vi "Reboot Target.vi"(8 "Error In":errorcluster, 11 "Install LV Data":T1={"SSH Session"=refnum, "Status Log"="", "Detailed Log"="", "Credentials"={"Hostname or IP"="192.168.7.2", "Username"="root", "Password"=""}, "Target Info"={"OS Version"="", "CPU"="", "Systemd Version"="", "Internet Access"=FALSE, "Device Type"="", "LV Installed Ver"="", "LV Available Ver"="", "LV Upgrade Available"=FALSE, "Hostname"="", "NIC Info"=[]}, "Reboot Required?"=FALSE}) -> (0 "Error Out":errorcluster, 1 "Connected?":bool, 3 "Install LV Data":T1={"SSH Session"=refnum, "Status Log"="", "Detailed Log"="", "Credentials"={"Hostname or IP"="192.168.7.2", "Username"="root", "Password"=""}, "Target Info"={"OS Version"="", "CPU"="", "Systemd Version"="", "Internet Access"=FALSE, "Device Type"="", "LV Installed Ver"="", "LV Available Ver"="", "LV Upgrade Available"=FALSE, "Hostname"="", "NIC Info"=[]}, "Reboot Required?"=FALSE})   [LabVIEW 2020, in "LMH-LINX.lvlib"]
uses:
  LMH-LINX.lvlib
  Target Management/Install LV Data.ctl
  Target Management/Target Info.ctl
  Target Management/NIC Info.ctl
  Target Management/NIC Mode.ctl
panel:
  out "Reboot Error":errorcluster
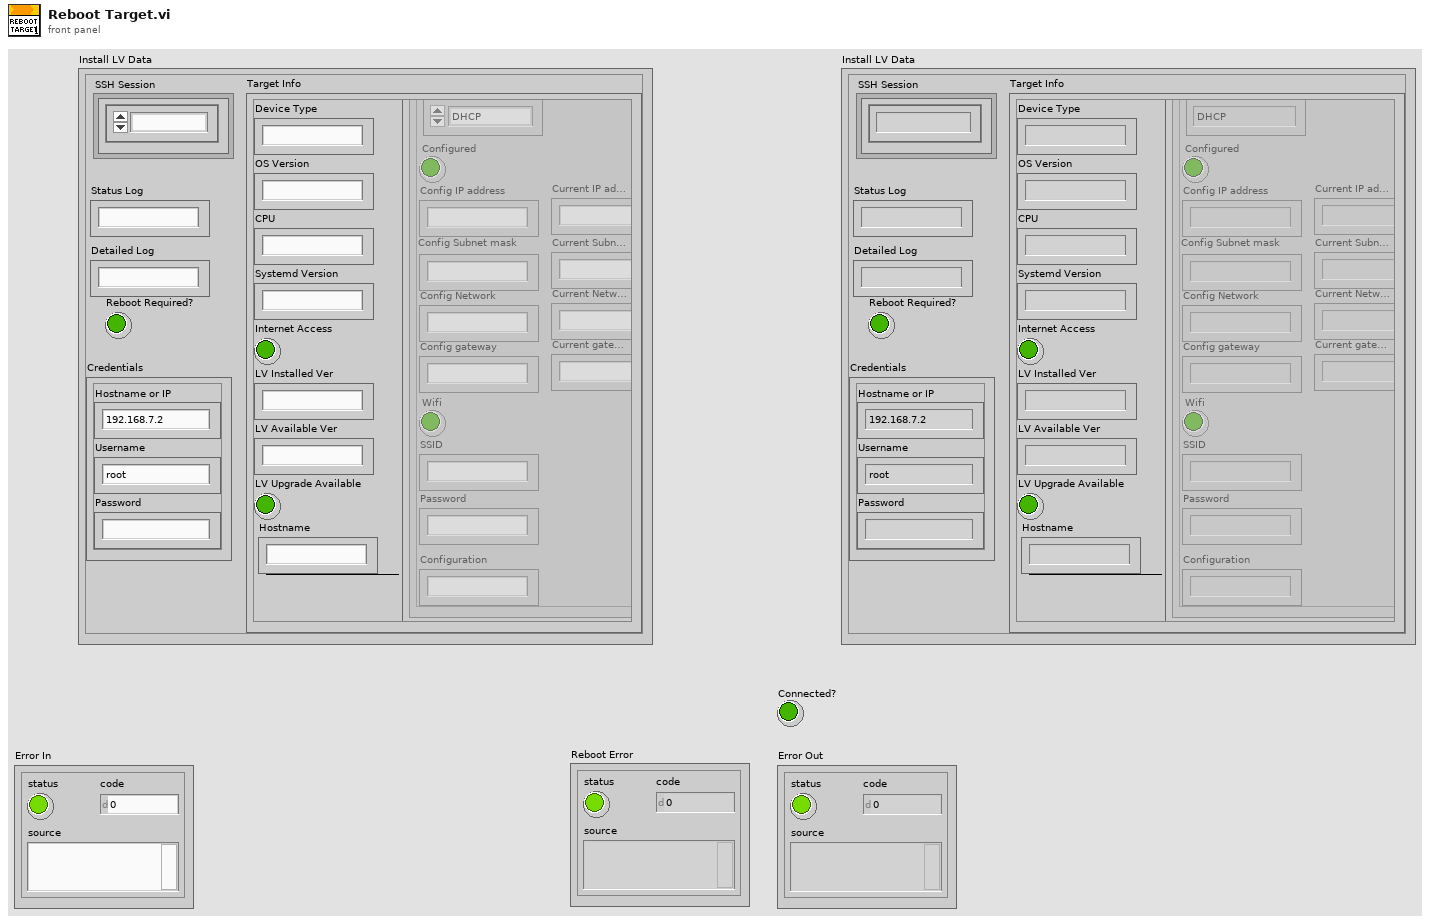
[diagram p1: front panel]
types:
  T1 = typedef "LMH-LINX.lvlib/Install LV Data.ctl" = cluster{"SSH Session":refnum<k1>, "Status Log":string, "Detailed Log":string, "Credentials":cluster{"Hostname or IP":string, "Username":string, "Password":string}, "Target Info":T2, "Reboot Required?":bool}
  T2 = typedef "LMH-LINX.lvlib/Target Info.ctl" = cluster{"OS Version":string, "CPU":string, "Systemd Version":string, "Internet Access":bool, "Device Type":string, "LV Installed Ver":string, "LV Available Ver":string, "LV Upgrade Available":bool, "Hostname":string, "NIC Info":T3[]}
  T3 = typedef "LMH-LINX.lvlib/NIC Info.ctl" = cluster{"Name":string, "NIC Mode":T4, "Configured":bool, "Config IP address":string, "Config Subnet mask":string, "Config Network":string, "Config gateway":string, "Wifi":bool, "SSID":string, "Password":string, "Configuration":string, "Current IP address":string, "Current Subnet mask":string, "Current gateway":string, "Current Network":string}
  T4 = typedef "LMH-LINX.lvlib/NIC Mode.ctl" = enum16{"DHCP", "Static", "Loopback"}
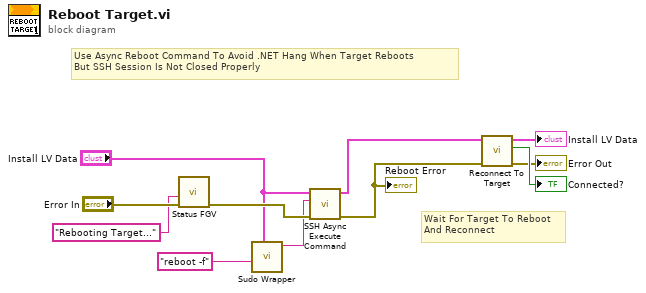
[diagram p0: block diagram]
diagram:
  # "Use Async Reboot Command To Avoid .NET Hang When Target Reboots \nBut SSH Session Is Not Closed Properly"
  # "Wait For Target To Reboot \nAnd Reconnect"
  n1 = call "Status FGV.vi"("Error In"="Error In", "Status"="Rebooting Target...") -> ("Error Out"=w7:errorcluster)  [unwired: 7 in, 2 out]
  n2 = call "Sudo Wrapper.vi"("Install LV Data"="Install LV Data", "comand string"="reboot -f" ("Command")) -> ("combined command string"=w2:string)  [unwired: 9 in]
  n3 = call "SSH Async Execute Command.vi"("Error In"=w7, "Command"=w2, "Install LV Data in"="Install LV Data") -> ("Error Out"=w5:errorcluster, "Install LV Data out"=w6:T1)  [unwired: 7 in]
  "Reboot Error" <- w5
  n4 = call "Reconnect To Target.vi"("Error In"=w5, "Install LV Data in"=w6) -> ("Error Out"=→"Error Out":errorcluster, "Connected?"=→"Connected?":bool, "Install LV Data out"=→"Install LV Data":T1)  [unwired: 7 in]
